vi "Read Next Message.vi"(8 "error in":errorcluster, 11 "Message queue":refnum<queue>) -> (0 "error out":errorcluster, 1 "Message Value":string, 2 "Message Name":string, 3 "Message queue out":refnum<queue>)   [LabVIEW 2021]
uses:
  Message.ctl
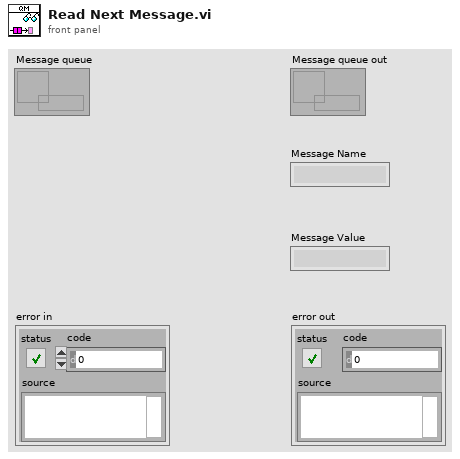
[diagram p1: front panel]
types:
  T1 = typedef "Message.ctl" = cluster{"Name":string, "Value":string, "Local IP":string, "Local Queue":string, "Remote IP":string, "Remote Queue":string}
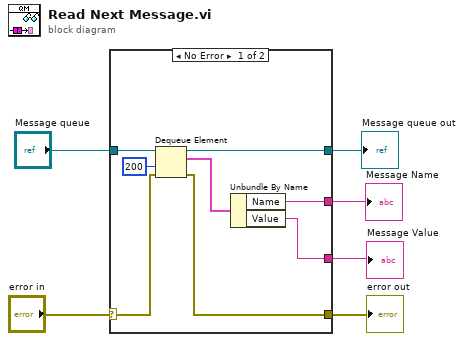
[diagram p0: block diagram]
diagram:
  n1 = case shown="No Error" "error in" {
    selector: "error in" -> [w13 w15]
    tunnel: "Message queue" -> [w14 w16]
    tunnel: [w8 w15] -> w4
    tunnel: [w12 w16] -> w5
    tunnel: [w10 _] -> w2
    tunnel: [w9 _] -> w1
    frame No Error {
      n2 = Dequeue Element(queue=w14, timeout in ms (-1)=200, error in (no error)=w13) -> (queue out=w12:refnum<queue>, element=w11:T1, error out=w8:errorcluster)  [unwired: 1 out]
      n3 = Unbundle By Name(w11) -> ("Name"=w10:string, "Value"=w9:string)
    }
    frame Error {
    }
  }
  "error out" <- w4
  "Message queue out" <- w5
  "Message Name" <- w2
  "Message Value" <- w1
